vi "Create Move Axis Commands.vi"() -> ()   [LabVIEW 2019, in "XYStage.KIM101.lvclass"]
uses:
  XYStage.KIM101.lvclass
panel:
  in  "Axis":string
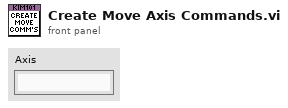
[diagram p1: front panel]
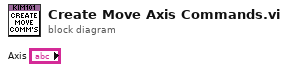
[diagram p0: block diagram]
diagram:
